vi "sv_Build dB Label (octave info).vi"(4 "width (-)":i16, 5 "number format":i16(ring) items=["Engineering", "Exponential", "Fractional", "Automatic"], 7 "include reference (T)":bool=TRUE, 8 "error in (no error)":errorcluster, 9 "precision (1)":i16=1, 10 "octave info":T1={"standard"=enum."ANSI S1.11", "bandwidth"=enum."1 octave", "low band"=0, "high band"=0, "weighting filter"=0, "dB reference"=0.0, "dB On"=FALSE, "unit label"="", "channel name"="", "description"="", "engineering units"=1, "custom label"="", "spectrum type"=enum."magnitude", "spectral density"=FALSE, "filters settled"=FALSE} {"engineering units" items=["custom..."=0, "V"=1, "A"=21, "C"=30, "pC"=31, "s"=32, "-"=29, "Pa"=2, "N"=20, "g"=3, "m/s^2"=4, "m/s"=5, "m"=6, "mm/s"=12, "mm"=13, "micron/s"=14, "micron"=15, "in/s^2"=7, "in/s"=8, "in"=9, "mil/s"=10, "mil"=11, "rad/s^2"=16, "rad/s"=17, "rad"=18, "deg/s^2"=26, "deg/s"=27, "deg"=28, "RPM"=22, "cycle/s^2"=23, "Hz"=24, "cycle"=25, "strain"=19]; "dB reference" format="%.2e"; "weighting filter" items=["Linear", "A-weighting", "B-weighting", "C-weighting", "ITU-R 468-4", "Dolby", "CCITT", "C-message", "Wb", "Wc", "Wd", "We", "Wf", "Wh", "Wj", "Wk", "Wm", "AES17 20 kHz lowpass", "AES17 40 kHz lowpass", "AES17 20 kHz highpass", "AES17 40 kHz highpass"]}) -> (0 "error out":errorcluster, 1 "dB reference [EU]":dbl format="%.2f", 2 "ref label":string, 3 "dB( )":string)   [LabVIEW 2017, in "SoundVib_Octave_2014 standard.lvlib"]
uses:
  <vilib>/addons/Sound and Vibration/svt_Octave/SoundVib_Octave_2014 standard.lvlib
  <vilib>/addons/_NISVFA/_Shared subVIs/Controls/svc_Octave Info.ctl
  <vilib>/addons/_NISVFA/_Shared subVIs/Controls/svc_Octave Standard.ctl
  <vilib>/addons/_NISVFA/_Shared subVIs/Controls/svc_Weighting Filter Text Ring.ctl
  <vilib>/addons/_NISVFA/_Shared subVIs/Controls/svc_Engineering Units Text Ring.ctl
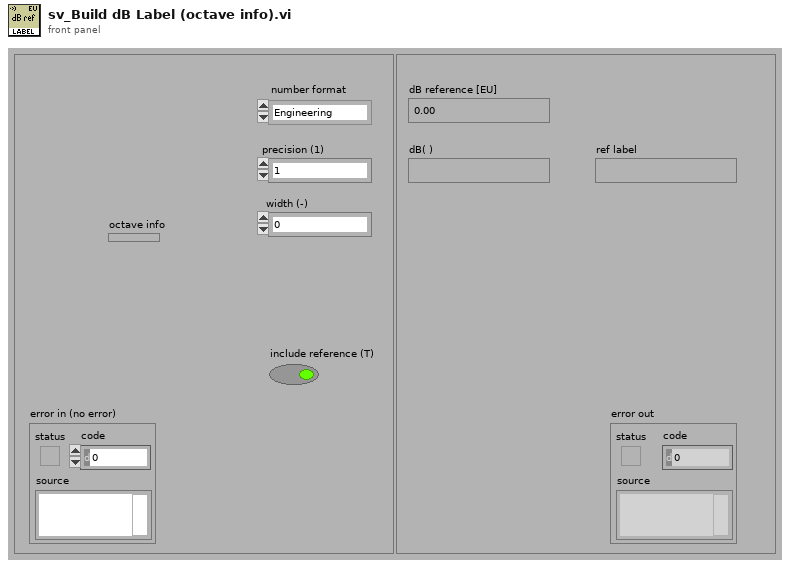
[diagram p1: front panel]
types:
  T1 = typedef "svc_Octave Info.ctl" = cluster{"standard":T2, "bandwidth":enum16{"1 octave", "1/3 octave", "1/6 octave", "1/12 octave", "1/24 octave"}, "low band":i32, "high band":i32, "weighting filter":T3, "dB reference":dbl, "dB On":bool, "unit label":string, "channel name":string, "description":string, "engineering units":T4, "custom label":string, "spectrum type":enum16{"power", "magnitude"}, "spectral density":bool, "filters settled":bool}
  T2 = typedef "svc_Octave Standard.ctl" = enum16{"ANSI S1.11", "IEC 61260"}
  T3 = typedef "svc_Weighting Filter Text Ring.ctl" = u16
  T4 = typedef "svc_Engineering Units Text Ring.ctl" = u16
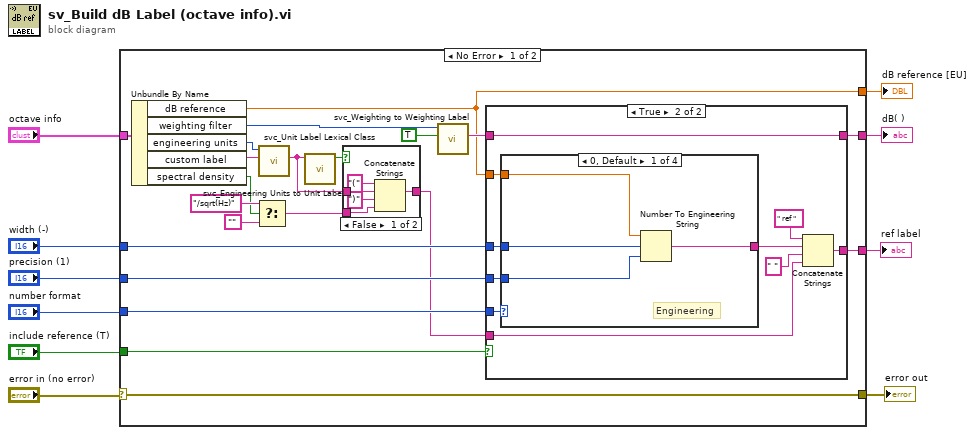
[diagram p0: block diagram]
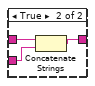
[diagram p2: hidden frame]
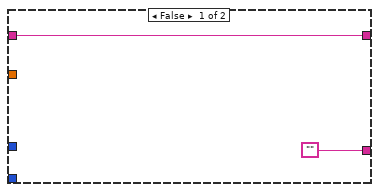
[diagram p3: hidden frame]
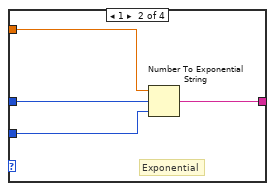
[diagram p4: hidden frame]
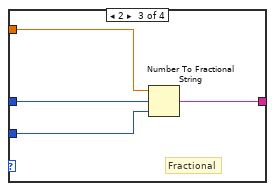
[diagram p5: hidden frame]
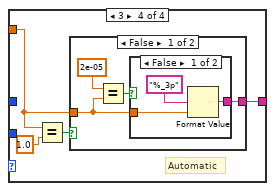
[diagram p6: hidden frame]
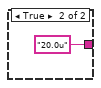
[diagram p7: hidden frame]
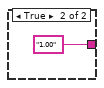
[diagram p8: hidden frame]
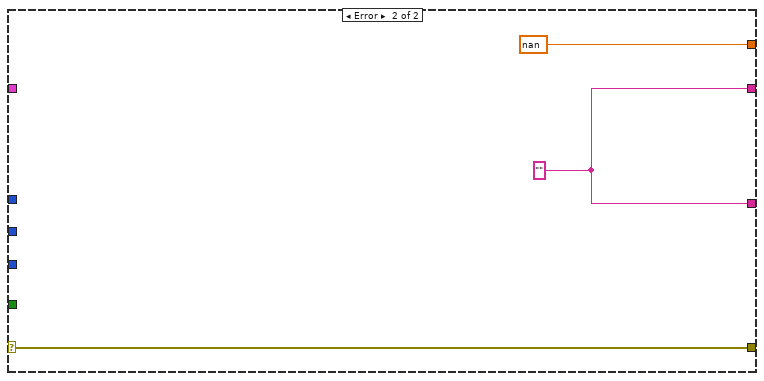
[diagram p9: hidden frame]
diagram:
  n1 = case shown="No Error" "error in (no error)" {
    selector: "error in (no error)" -> [w29 w79]
    tunnel: "include reference (T)" -> [w31 _]
    tunnel: "octave info" -> [w27 _]
    tunnel: [w30 w78] -> w7
    tunnel: [w29 w79] -> w6
    tunnel: "number format" -> [w28 _]
    tunnel: [w24 w78] -> w4
    tunnel: [w20 nan ("dB reference [EU]")] -> w3
    tunnel: "width (-)" -> [w22 _]
    tunnel: "precision (1)" -> [w21 _]
    frame No Error {
      n2 = Unbundle By Name(w27) -> ("dB reference"=w20:dbl, "weighting filter"=w26:T3, "engineering units"=w17:T4, "custom label"=w16:string, "spectral density"=w12:bool)
      n3 = Select(t="/sqrt(Hz)", s=w12, f="") -> (s? t:f=w13:string)
      n4 = call <vilib>:"svc_Engineering Units to Unit Label.vi"("custom label"=w16, "engineering units"=w17) -> ("unit label"=w19:string)  [unwired: 8 in, 1 out]
      n5 = call <vilib>:"svc_Unit Label Lexical Class.vi"("unit label"=w19) -> ("letters only?"=w18:bool)  [unwired: 6 in]
      n6 = case shown="False" w18 {
        tunnel: w19 -> [w36 w39]
        tunnel: [w35 w37] -> w15
        tunnel: w13 -> [w32 w38]
        frame False {
          n7 = Concatenate Strings("(" ("string"), w36, ")" ("string"), w32) -> (w35:string)
        }
        frame True {
          n8 = Concatenate Strings(w39, w38) -> (w37:string)
        }
      }
      n9 = call <vilib>:"svc_Weighting to Weighting Label.vi"("dB On (T)"=TRUE, "weighting filter"=w26) -> ("weighting string"=w25:string)  [unwired: 8 in, 1 out]
      n10 = case shown="True" w31 {
        tunnel: ["" w51] -> w30
        tunnel: w20 -> [_ w46]
        tunnel: w28 -> [_ w44]
        tunnel: w15 -> [_ w49]
        tunnel: [w40 w47] -> w24
        tunnel: w25 -> [w40 w47]
        tunnel: w22 -> [_ w43]
        tunnel: w21 -> [_ w42]
        frame False {
        }
        frame True {
          n11 = case shown="0, Default" w44 {
            tunnel: [w53 w59 w63 w67] -> w45
            tunnel: w43 -> [w54 w58 w62 _]
            tunnel: w42 -> [w55 w57 w61 _]
            tunnel: w46 -> [w52 w56 w60 w66]
            frame 0, Default {
              # "Engineering"
              n12 = Number To Engineering String(2:w55, 3:w54, 4:w52) -> (0:w53:string)  [unwired: 1 in]
            }
            frame 1 {
              # "Exponential"
              n13 = Number To Exponential String(number=w56, precision (6)=w57, 3:w58) -> (E-format string=w59:string)  [unwired: 1 in]
            }
            frame 2 {
              # "Fractional"
              n14 = Number To Fractional String(number=w60, width (-)=w62, precision (6)=w61) -> (F-format string=w63:string)  [unwired: 1 in]
            }
            frame 3 {
              # "Automatic"
              n15 = Equal?(x=w66, y=1.0) -> (x = y?=w64:bool)
              n16 = case shown="False" w64 {
                tunnel: [w71 "1.00" ("format string")] -> w67
                tunnel: w66 -> [w70 _]
                frame False {
                  n17 = Equal?(x=2e-05 ("y"), y=w70) -> (x = y?=w68:bool)
                  n18 = case shown="False" w68 {
                    tunnel: [w73 "20.0u" ("format string")] -> w71
                    tunnel: w70 -> [w72 _]
                    frame False {
                      n19 = Format Value(format string="%_3p", value (0)=w72) -> (output string=w73:string)  [unwired: 1 in]
                    }
                    frame True {
                    }
                  }
                }
                frame True {
                }
              }
            }
          }
          n20 = Concatenate Strings(" ref ", w45, " " ("Substring"), w49) -> (w51:string)
        }
      }
    }
    frame Error {
      w78 = ""
    }
  }
  "error out" <- w6
  "ref label" <- w7
  "dB( )" <- w4
  "dB reference [EU]" <- w3
